vi "Generate Save Path.vi"(8 "error in (no error)":errorcluster, 11 "Log File Base Path":path) -> (0 "error out":errorcluster, 2 "Save String":string, 3 "Save Path":path)   [LabVIEW 2013, in "Logging.lvlib"]
uses:
  Logging.lvlib
  <vilib>/regexp/Match Regular Expression.xnode
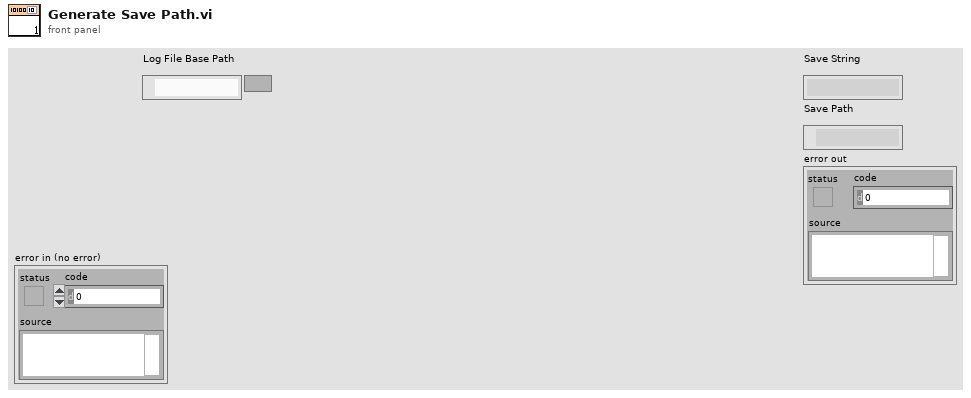
[diagram p1: front panel]
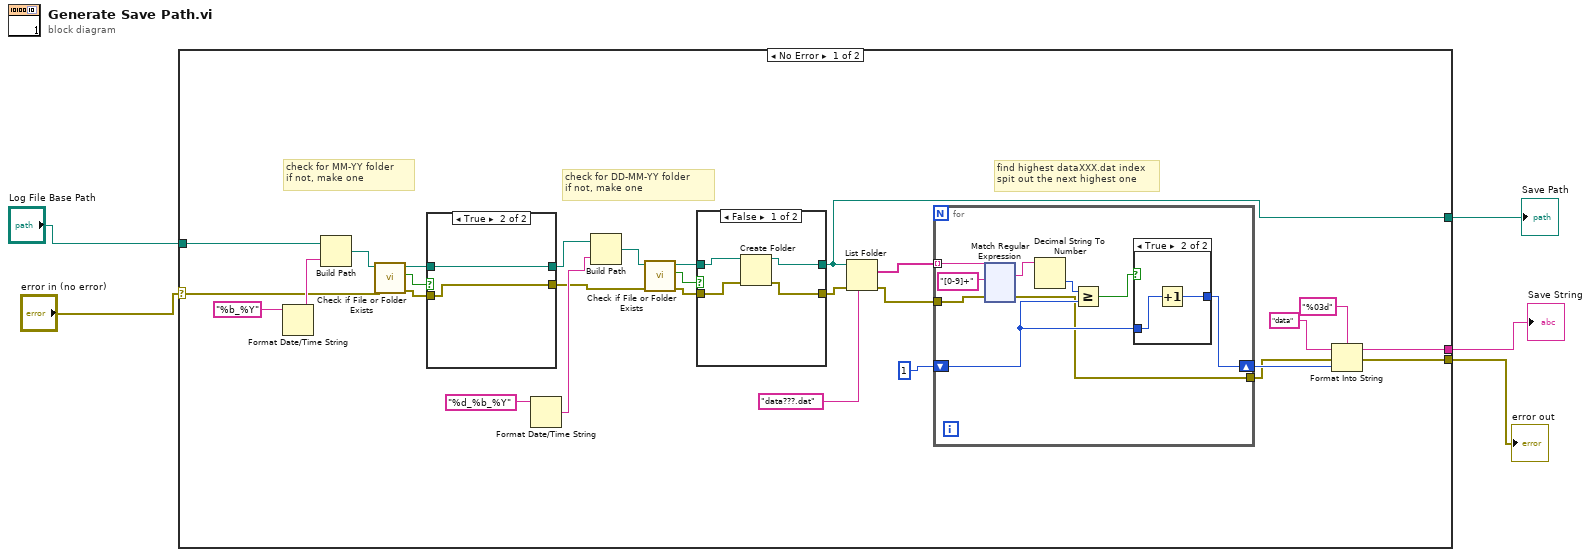
[diagram p0: block diagram]
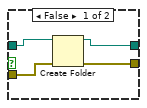
[diagram p4: hidden frame]
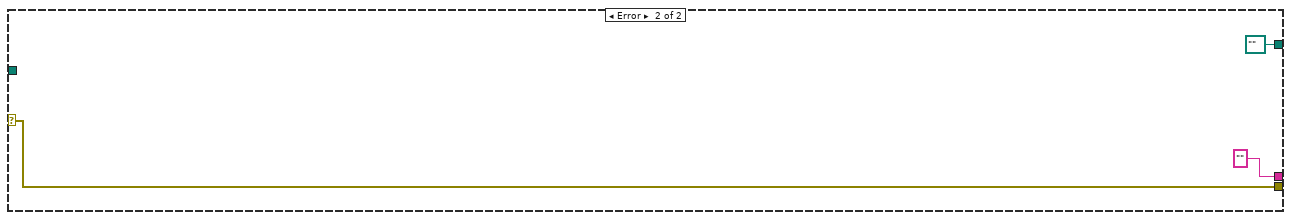
[diagram p5: hidden frame]
diagram:
  n1 = case shown="No Error" "error in (no error)" {
    selector: "error in (no error)" -> [w8 w174]
    tunnel: [w19 path "" ("dup path")] -> w5
    tunnel: [w10 ""] -> w4
    tunnel: "Log File Base Path" -> [w9 _]
    tunnel: [w6 w174] -> w1
    frame No Error {
      # "find highest dataXXX.dat index\nspit out the next highest one"
      # "check for DD-MM-YY folder\nif not, make one"
      # "check for MM-YY folder\nif not, make one"
      n2 = Format Date/Time String(time format string (%c)="%b_%Y") -> (date/time string=w31:string)  [unwired: 2 in]
      n3 = Build Path(base path=w9, name or relative path=w31) -> (appended path=w29:path)
      n4 = call <vilib>:"Check if File or Folder Exists.vi"("error in (no error)"=w8, "path"=w29) -> ("error out"=w27:errorcluster, "file or folder exists?"=w30:bool, "dup path"=w28:path)  [unwired: 7 in]
      n5 = case shown="True" w30 {
        tunnel: [w168 w171] -> w22
        tunnel: w28 -> [w169 w171]
        tunnel: w27 -> [w167 w170]
        tunnel: [w166 w170] -> w20
        frame False {
          n6 = Create Folder(path (use dialog)=w169, error in=w167) -> (created path=w168:path, error out=w166:errorcluster)  [unwired: 1 in, 1 out]
        }
        frame True {
        }
      }
      n7 = Format Date/Time String(time format string (%c)="%d_%b_%Y") -> (date/time string=w21:string)  [unwired: 2 in]
      n8 = Build Path(base path=w22, name or relative path=w21) -> (appended path=w25:path)
      n9 = call <vilib>:"Check if File or Folder Exists.vi"("error in (no error)"=w20, "path"=w25) -> ("error out"=w23:errorcluster, "file or folder exists?"=w26:bool, "dup path"=w24:path)  [unwired: 7 in]
      n10 = case shown="False" w26 {
        tunnel: [w162 w165] -> w19
        tunnel: w24 -> [w163 w165]
        tunnel: w23 -> [w161 w164]
        tunnel: [w160 w164] -> w17
        frame False {
          n11 = Create Folder(path (use dialog)=w163, error in=w161) -> (created path=w162:path, error out=w160:errorcluster)  [unwired: 1 in, 1 out]
        }
        frame True {
        }
      }
      n12 = List Folder(path=w19, pattern="data???.dat" ("time format string (%c)"), error in=w17) -> (filenames=w16:string[], error out=w15:errorcluster)  [unwired: 1 in, 2 out]
      n13 = for {
        tunnel: w16 -> [w42] mode=indexing
        tunnel: w15 -> [w41]
        shift-right: [w37] -> w12
        shift-left: 1 ("number") -> [w36]
        tunnel: [w35] -> w7
        n14 = xnode "Match Regular Expression"("input string"=w42, "regular expression"="[0-9]+", "error in"=w41) -> ("whole match"=w34:string, "error out"=w35:errorcluster)  [unwired: 3 in, 3 out]
        n15 = Decimal String To Number(string=w34) -> (number=w39:i32)  [unwired: 2 in, 1 out]
        n16 = Greater Or Equal?(x=w39, y=w36) -> (x >= y?=w38:bool)
        n17 = case shown="True" w38 {
          tunnel: w36 -> [w43 w45]
          tunnel: [w43 w44] -> w37
          frame False {
          }
          frame True {
            n18 = Increment(x=w45) -> (x+1=w44:i32)
          }
        }
      }
      n19 = Format Into String(format string="%03d", initial string="data" ("time format string (%c)"), error in=w7, w12) -> (resulting string=w10:string, error out=w6:errorcluster)
    }
    frame Error {
    }
  }
  "Save String" <- w4
  "Save Path" <- w5
  "error out" <- w1
